vi "LTE Common Configure.vi"(0 "Instrument Handle In":refnum<k21>, 1 "Selector String":string, 5 "Common Configuration":T1={"Center Frequency (Hz)"=1000000000.0, "Reference Level (dBm)"=0.0, "External Attenuation (dB)"=0.0, "Frequency Reference Source"="OnboardClock", "Enable Trigger?"=TRUE, "Digital Edge Source"="PXI_Trig0", "Digital Edge"=0, "Trigger Delay (s)"=0.0} {"External Attenuation (dB)" format="%.2f"; "Reference Level (dBm)" format="%.2f"; "Center Frequency (Hz)" format="%.6p"; "Trigger Delay (s)" format="%.3p"; "Digital Edge" items=["Rising Edge", "Falling Edge"]}, 11 "error in (no error)":errorcluster) -> (4 "Instrument Handle Out":refnum<k21>, 15 "error out":errorcluster)   [LabVIEW 2018, in "RFmxLTE.lvlib"]
uses:
  RFmxLTE.lvlib
  Typedefs/LTE Common Configuration.ctl
  <vilib>/RFmx/LTE/mx/RFmxLTE.llb/RFmxLTE Configure Digital Edge Trigger.vi
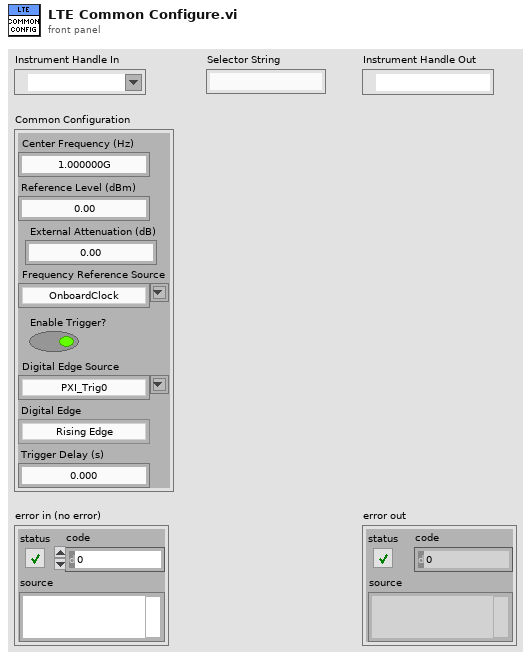
[diagram p1: front panel]
types:
  T1 = typedef "RFmxLTE.lvlib/LTE Common Configuration.ctl" = cluster{"Center Frequency (Hz)":dbl, "Reference Level (dBm)":dbl, "External Attenuation (dB)":dbl, "Frequency Reference Source":string, "Enable Trigger?":bool, "Digital Edge Source":string, "Digital Edge":i32, "Trigger Delay (s)":dbl}
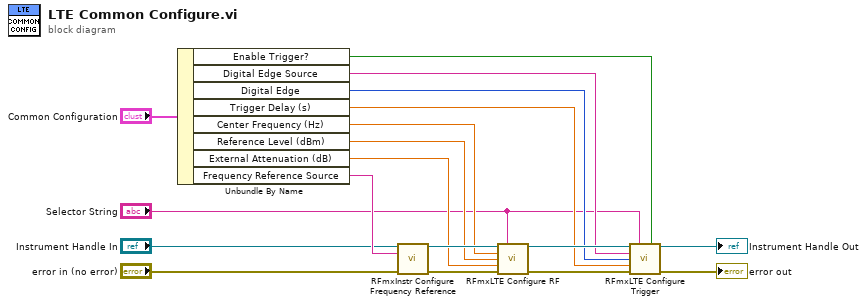
[diagram p0: block diagram]
diagram:
  n1 = Unbundle By Name("Common Configuration") -> ("Enable Trigger?"=w5:bool, "Digital Edge Source"=w8:string, "Digital Edge"=w7:i32, "Trigger Delay (s)"=w6:dbl, "Center Frequency (Hz)"=w11:dbl, "Reference Level (dBm)"=w12:dbl, "External Attenuation (dB)"=w13:dbl, "Frequency Reference Source"=w16:string)
  n2 = call <vilib>:"RFmxInstr Configure Frequency Reference.vi"("Instrument Handle In"="Instrument Handle In", "Frequency Reference Source"=w16, "error in (no error)"="error in (no error)") -> ("Instrument Handle Out"=w15:refnum<k21>, "error out"=w14:errorcluster)  [unwired: 11 in]
  n3 = call <vilib>:"RFmxLTE Configure RF.vi"("Instrument Handle In"=w15, "Selector String"="Selector String", "Center Frequency (Hz)"=w11, "Reference Level"=w12, "External Attenuation (dB)"=w13, "error in (no error)"=w14) -> ("Instrument Handle Out"=w10:refnum<k21>, "error out"=w9:errorcluster)  [unwired: 8 in]
  n4 = call-poly <vilib>:"RFmxLTE Configure Trigger.vi"("Instrument Handle In"=w10, "Selector String"="Selector String", "Enable Trigger?"=w5, "Digital Edge Source"=w8, "Digital Edge"=w7, "Trigger Delay (s)"=w6, "error in (no error)"=w9) -> ("Instrument Handle Out"=→"Instrument Handle Out":refnum<k21>, "error out"=→"error out":errorcluster)  [unwired: 7 in]
